vi "BCDaSS.vi"(1 "D":bool, 2 "C":bool, 3 "B":bool, 4 "A":bool) -> (0 "display":T1)   [LabVIEW 2016]
doc: "Este subVI es una herramienta que nos ayudara a la visualización grafica de números en un display, números que van del 0 al 9."
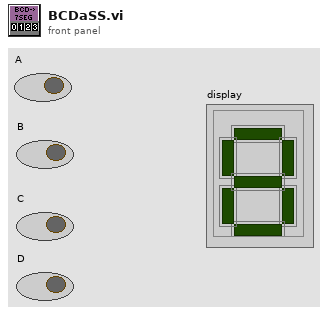
[diagram p1: front panel]
types:
  T1 = cluster{"A":bool, "B":bool, "C":bool, "E":bool, "D":bool, "F":bool, "G":bool}
  T2 = cluster{bool, bool, bool, bool, bool, bool, bool}
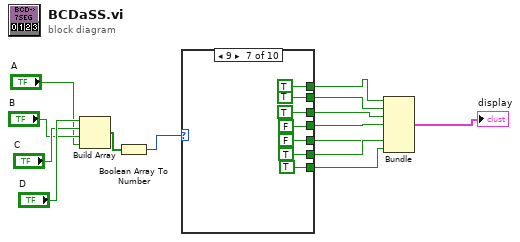
[diagram p0: block diagram]
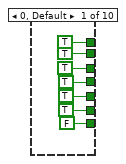
[diagram p2: hidden frame]
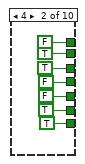
[diagram p3: hidden frame]
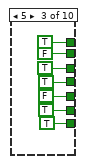
[diagram p4: hidden frame]
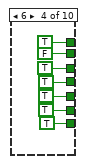
[diagram p5: hidden frame]
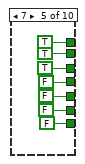
[diagram p6: hidden frame]
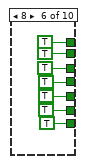
[diagram p7: hidden frame]
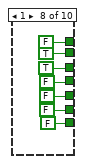
[diagram p8: hidden frame]
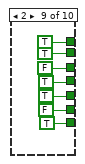
[diagram p9: hidden frame]
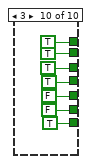
[diagram p10: hidden frame]
diagram:
  n1 = Build Array("D", "C", "B", "A") -> (w5:bool[])
  n2 = Boolean Array To Number(Boolean array=w5) -> (number=w6:u32)
  n3 = case shown="9" w6 {
    tunnel: [TRUE FALSE TRUE TRUE TRUE TRUE TRUE FALSE TRUE TRUE] -> w8
    tunnel: [TRUE TRUE FALSE FALSE TRUE TRUE TRUE TRUE TRUE TRUE] -> w9
    tunnel: [TRUE TRUE TRUE TRUE TRUE TRUE TRUE TRUE FALSE TRUE] -> w10
    tunnel: [TRUE FALSE TRUE TRUE FALSE TRUE FALSE FALSE TRUE TRUE] -> w11
    tunnel: [TRUE FALSE FALSE TRUE FALSE TRUE FALSE FALSE TRUE FALSE] -> w12
    tunnel: [TRUE TRUE TRUE TRUE FALSE TRUE TRUE FALSE FALSE FALSE] -> w13
    tunnel: [FALSE TRUE TRUE TRUE FALSE TRUE TRUE FALSE TRUE TRUE] -> w14
    frame 0, Default {
    }
    frame 4 {
    }
    frame 5 {
    }
    frame 6 {
    }
    frame 7 {
    }
    frame 8 {
    }
    frame 9 {
    }
    frame 1 {
    }
    frame 2 {
    }
    frame 3 {
    }
  }
  n4 = Bundle(w8, w9, w10, w11, w12, w13, w14) -> (→"display":T2)  [unwired: 1 in]
